vi "dataBuffer.vi"(6 "command":T2=enum."read recent", 8 "error in (no error)":errorcluster, 10 "max array size":u16=5000 min=1, 11 "averaged data":T1) -> (0 "error out":errorcluster, 1 "recent time":timestamp, 2 "scans":i32, 3 "recent data":dbl[](array[numeric]), 5 "misc graph":cluster{timestamp[], dbl[]}[](graph), 7 "turbidity":cluster{timestamp[], dbl[]}[](graph))   [LabVIEW 2015]
uses:
  Sensor buffer command.ctl
  data array with time.ctl
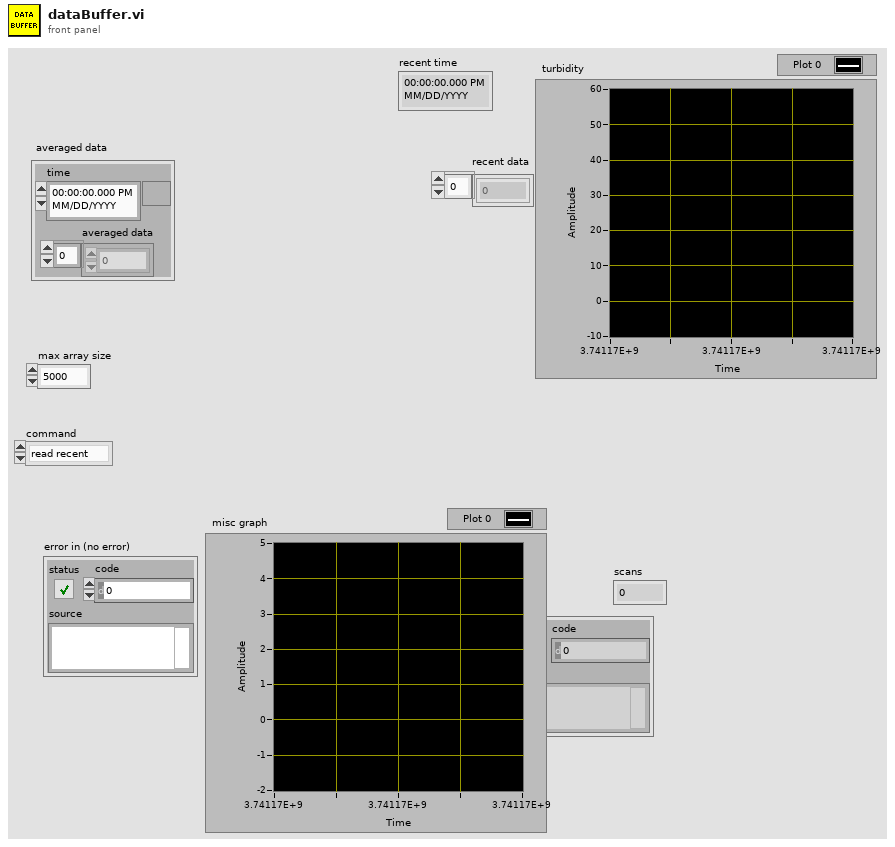
[diagram p1: front panel]
types:
  T1 = typedef "data array with time.ctl" = cluster{"time":timestamp, "averaged data":dbl[]}
  T2 = typedef "Sensor buffer command.ctl" = enum16{"set buffer size", "write", "refill buffer", "read recent", "read all", "clear"}
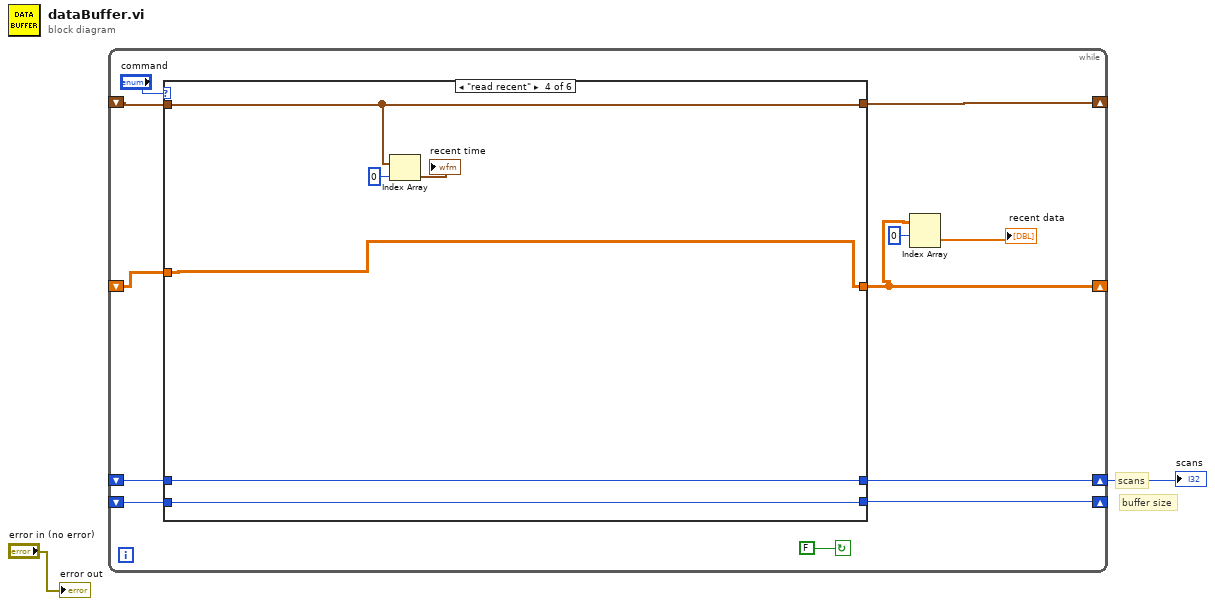
[diagram p0: block diagram]
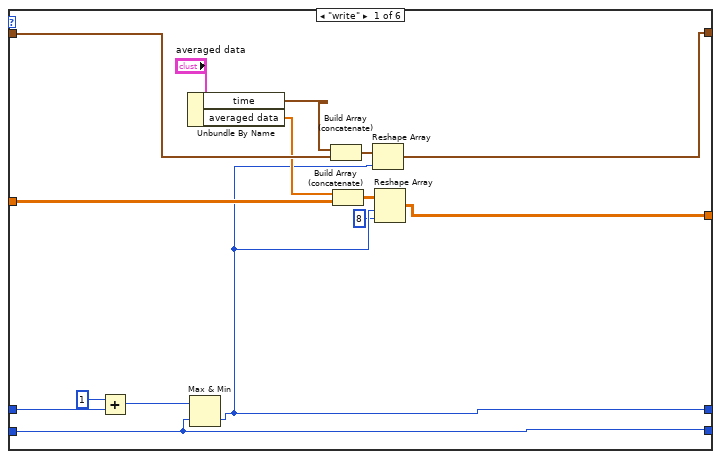
[diagram p2: hidden frame]
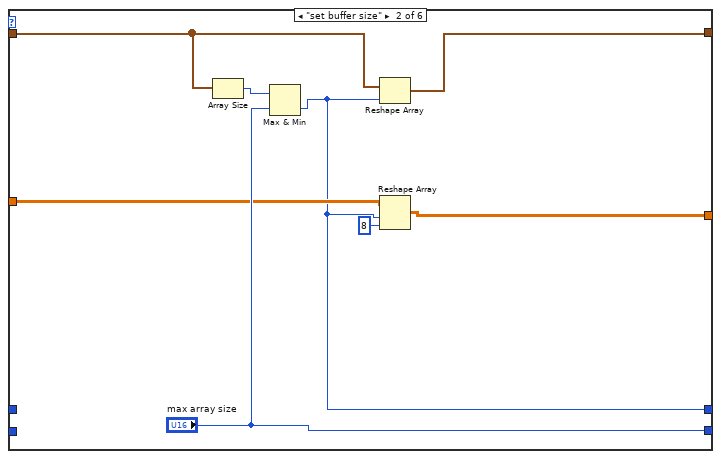
[diagram p3: hidden frame]
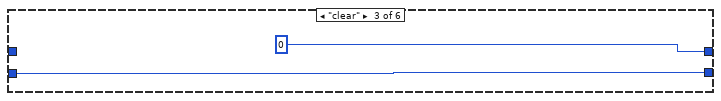
[diagram p4: hidden frame]
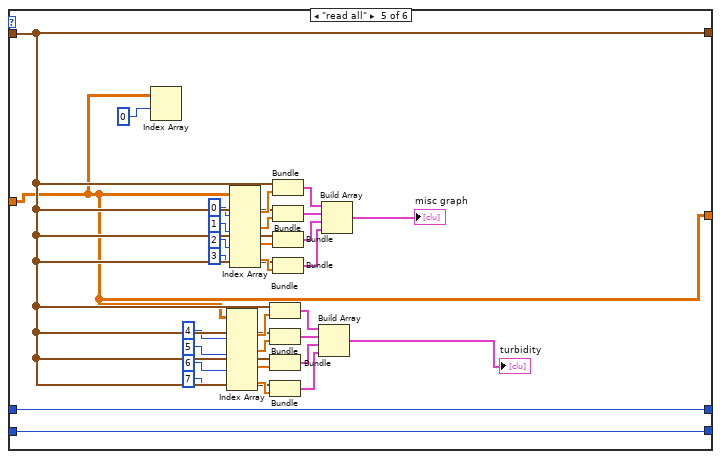
[diagram p5: hidden frame]
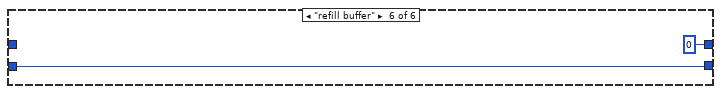
[diagram p6: hidden frame]
diagram:
  # "buffer size"
  # "scans"
  n1 = while {
    shift-right: [w13] -> _
    shift-left: _ -> [w12]
    shift-right: [w11] -> _
    shift-left: _ -> [w10]
    shift-right: [w7] -> w1
    shift-left: _ -> [w8]
    shift-right: [w3] -> _
    shift-left: _ -> [w6]
    stop <- FALSE continue-if-true
    n2 = case shown="\"read recent\"" "command" {
      tunnel: [w26 w37 _ w42 w56 _] -> w13
      tunnel: w12 -> [w28 w36 _ w42 w56 _]
      tunnel: [w24 "max array size" w39 w45 w76 w78] -> w11
      tunnel: w10 -> [w24 _ w39 w45 w76 w78]
      tunnel: w8 -> [w27 _ _ w44 w75 _]
      tunnel: [w16 w31 0 w44 w75 0] -> w7
      tunnel: [w18 w32 _ w40 w47 _] -> w3
      tunnel: w6 -> [w17 w33 _ w40 w47 _]
      frame "write" {
        n3 = Add(x=1, y=w27) -> (x+y=w23:i32)
        n4 = Unbundle By Name("averaged data") -> ("time"=w21:timestamp, "averaged data"=w19:dbl[])
        n5 = Max & Min(x=w23, y=w24) -> (min(x,y)=w16:i32)  [unwired: 1 out]
        n6 = Build Array (concatenate)(w21, w28) -> (w25:timestamp[])
        n7 = Build Array (concatenate)(w19, w17) -> (w20:dbl[][])
        n8 = Reshape Array(w25, w16) -> (w26:timestamp[])
        n9 = Reshape Array(w20, w16, 8 ("dimension size")) -> (w18:dbl[][])
      }
      frame "set buffer size" {
        n10 = Array Size(array=w36) -> (size(s)=w35:i32)
        n11 = Max & Min(x=w35, y="max array size") -> (min(x,y)=w31:i32)  [unwired: 1 out]
        n12 = Reshape Array(w36, w31) -> (w37:timestamp[])
        n13 = Reshape Array(w33, w31, 8 ("dimension size")) -> (w32:dbl[][])
      }
      frame "clear" {
      }
      frame "read recent" {
        n14 = Index Array(array=w42, index=0) -> (element=→"recent time":timestamp)
      }
      frame "read all" {
        n15 = Index Array(array=w47, index (row)=0) -> ()  [unwired: 1 in, 1 out]
        n16 = Index Array(array=w47, index (col) #1=4 ("index (row)"), index (col) #2=5 ("index (row)"), index (col) #3=6 ("index (row)"), index (col) #4=7 ("index (row)")) -> (element #1=w58:dbl[], element #2=w59:dbl[], element #3=w60:dbl[], element #4=w61:dbl[])  [unwired: 4 in]
        n17 = Index Array(array=w47, index (col) #1=0 ("index (row)"), index (col) #2=1 ("index (row)"), index (col) #3=2 ("index (row)"), index (col) #4=3 ("index (row)")) -> (element #1=w74:dbl[], element #2=w73:dbl[], element #3=w72:dbl[], element #4=w71:dbl[])  [unwired: 4 in]
        n18 = Bundle(w56, w58) -> (w62:cluster{timestamp[], dbl[]})  [unwired: 1 in]
        n19 = Bundle(w56, w59) -> (w63:cluster{timestamp[], dbl[]})  [unwired: 1 in]
        n20 = Bundle(w56, w60) -> (w64:cluster{timestamp[], dbl[]})  [unwired: 1 in]
        n21 = Bundle(w56, w61) -> (w65:cluster{timestamp[], dbl[]})  [unwired: 1 in]
        n22 = Bundle(w56, w74) -> (w70:cluster{timestamp[], dbl[]})  [unwired: 1 in]
        n23 = Bundle(w56, w73) -> (w69:cluster{timestamp[], dbl[]})  [unwired: 1 in]
        n24 = Bundle(w56, w72) -> (w67:cluster{timestamp[], dbl[]})  [unwired: 1 in]
        n25 = Bundle(w56, w71) -> (w66:cluster{timestamp[], dbl[]})  [unwired: 1 in]
        n26 = Build Array(w62, w63, w64, w65) -> (→"turbidity":cluster{timestamp[], dbl[]}[])
        n27 = Build Array(w70, w69, w67, w66) -> (→"misc graph":cluster{timestamp[], dbl[]}[])
      }
      frame "refill buffer" {
      }
    }
    n28 = Index Array(array=w3, index (row)=0 ("index")) -> (element=→"recent data":dbl[])  [unwired: 1 in]
  }
  "scans" <- w1
  "error out" <- "error in (no error)"
